vi "Miso Logic 256-bit.vi"(0 "MISO":bool, 5 "sample MISO":bool, 7 "controller interface":T1) -> (4 "read data":bool[](array[boolean]))   [LabVIEW 2015, in "SPI API.lvlib"]
doc: "This VI captures a single bit of MISO data to for the read data word."
uses:
  Controls/Controller Interface.ctl
  SPI API.lvlib
panel:
  # "This VI captures a single bit of MISO data to for the read data word."
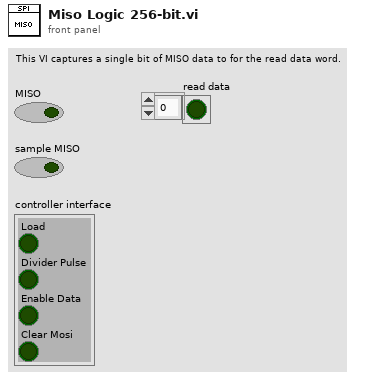
[diagram p1: front panel]
types:
  T1 = typedef "SPI API.lvlib/Controller Interface.ctl" = cluster{"Load":bool, "Divider Pulse":bool, "Enable Data":bool, "Clear Mosi":bool}
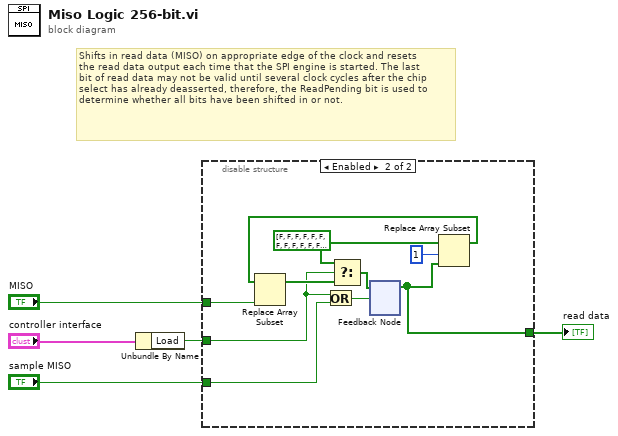
[diagram p0: block diagram]
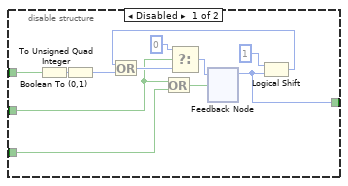
[diagram p2: hidden frame]
diagram:
  # "Shifts in read data (MISO) on appropriate edge of the clock and resets\nthe read data output each time that the SPI engine is started. The last\nbit of read data may not be valid until several clock cycles after the chip select has already deasserted, therefore, the ReadPending bit is used to determine whether all bits have been shifted in or not."
  n1 = Unbundle By Name("controller interface") -> ("Load"=w5:bool)
  n2 = disable-structure shown="Enabled" {
    disable-tunnel: [w16 w18] -> w1
    disable-tunnel: "MISO" -> [w7 w22]
    disable-tunnel: w5 -> [w10 w23]
    disable-tunnel: "sample MISO" -> [w9 w25]
    frame Disabled {
      n3 = Boolean To (0,1)(Boolean=w7) -> (0, 1=w6:i16)
      n4 = To Unsigned Quad Integer(1:w6) -> (0:w8:u64)
      n5 = Or(x=w10, y=w9) -> (x .or. y?=w14:bool)
      n6 = feedback #1() -> (w16:u64)  [unwired: 1 in]
      n7 = Logical Shift(y=i16 1, x=w16) -> (x << y=w15:u64)
      n8 = Or(x=w15, y=w8) -> (x .or. y?=w13:u64)
      n9 = Select(t=u64 0, s=w10, f=w13) -> (s? t:f=w12:u64)
      n10 = feedback-in #1(w12, w14) -> ()
    }
    frame Enabled {
      w21 = bool[] [FALSE, FALSE, FALSE, FALSE, FALSE, FALSE, FALSE, FALSE, FALSE, FALSE, FALSE, FALSE, FALSE, FALSE, FALSE, FALSE, FALSE, FALSE, FALSE, FALSE, FALSE, FALSE, FALSE, FALSE, FALSE, FALSE, FALSE, FALSE, FALSE, FALSE, FALSE, FALSE, FALSE, FALSE, FALSE, FALSE, FALSE, FALSE, FALSE, FALSE, FALSE, FALSE, FALSE, FALSE, FALSE, FALSE, FALSE, FALSE, FALSE, FALSE, FALSE, FALSE, FALSE, FALSE, FALSE, FALSE, FALSE, FALSE, FALSE, FALSE, FALSE, FALSE, FALSE, FALSE, FALSE, FALSE, FALSE, FALSE, FALSE, FALSE, FALSE, FALSE, FALSE, FALSE, FALSE, FALSE, FALSE, FALSE, FALSE, FALSE, FALSE, FALSE, FALSE, FALSE, FALSE, FALSE, FALSE, FALSE, FALSE, FALSE, FALSE, FALSE, FALSE, FALSE, FALSE, FALSE, FALSE, FALSE, FALSE, FALSE, FALSE, FALSE, FALSE, FALSE, FALSE, FALSE, FALSE, FALSE, FALSE, FALSE, FALSE, FALSE, FALSE, FALSE, FALSE, FALSE, FALSE, FALSE, FALSE, FALSE, FALSE, FALSE, FALSE, FALSE, FALSE, FALSE, FALSE, FALSE, FALSE, FALSE, FALSE, FALSE, FALSE, FALSE, FALSE, FALSE, FALSE, FALSE, FALSE, FALSE, FALSE, FALSE, FALSE, FALSE, FALSE, FALSE, FALSE, FALSE, FALSE, FALSE, FALSE, FALSE, FALSE, FALSE, FALSE, FALSE, FALSE, FALSE, FALSE, FALSE, FALSE, FALSE, FALSE, FALSE, FALSE, FALSE, FALSE, FALSE, FALSE, FALSE, FALSE, FALSE, FALSE, FALSE, FALSE, FALSE, FALSE, FALSE, FALSE, FALSE, FALSE, FALSE, FALSE, FALSE, FALSE, FALSE, FALSE, FALSE, FALSE, FALSE, FALSE, FALSE, FALSE, FALSE, FALSE, FALSE, FALSE, FALSE, FALSE, FALSE, FALSE, FALSE, FALSE, FALSE, FALSE, FALSE, FALSE, FALSE, FALSE, FALSE, FALSE, FALSE, FALSE, FALSE, FALSE, FALSE, FALSE, FALSE, FALSE, FALSE, FALSE, FALSE, FALSE, FALSE, FALSE, FALSE, FALSE, FALSE, FALSE, FALSE, FALSE, FALSE, FALSE, FALSE, FALSE, FALSE, FALSE, FALSE, FALSE, FALSE, FALSE, FALSE, FALSE, FALSE, FALSE, FALSE, FALSE, FALSE, FALSE, FALSE, FALSE, FALSE, FALSE, FALSE, FALSE, FALSE]
      n11 = Or(x=w23, y=w25) -> (x .or. y?=w27:bool)
      n12 = feedback #2() -> (w18:bool[])  [unwired: 1 in]
      n13 = Replace Array Subset(array=w21, new element=w18, index=1) -> (w19:bool[])
      n14 = Replace Array Subset(array=w19, new element=w22) -> (w24:bool[])  [unwired: 1 in]
      n15 = Select(t=w21, s=w23, f=w24) -> (s? t:f=w26:bool[])
      n16 = feedback-in #2(w26, w27) -> ()
    }
  }
  "read data" <- w1
